vi "Telescope HK Data to Table.vi"(10 "Ch Info":T1[](array[typedef]), 11 "HK Data Cluster":T3) -> (3 "Table":string[][](array[string]))   [LabVIEW 2021, in "Telescope.lvclass"]
uses:
  Telescope.lvclass
  hk-channel-class/HK Item/HK Channel cluster Telemetry Data.ctl
  hk-channel-class/HK Item/HK Channel enum Data Type.ctl
  hk-channel-class/HK Item/HK Channel Units and Setup.ctl
  hk-channel-class/HK Item/HK Item.lvclass
panel:
  in  "Housekeeping Data":i32(listbox)
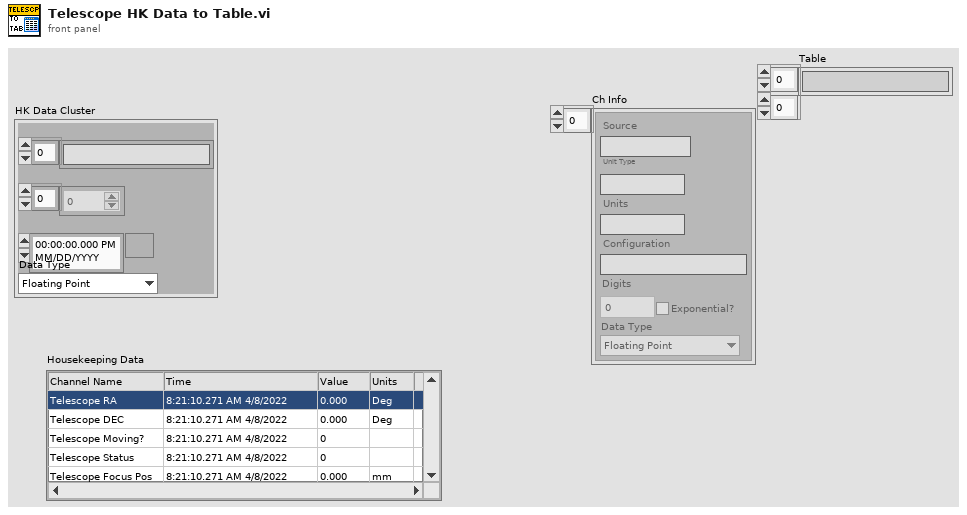
[diagram p1: front panel]
types:
  T1 = typedef "HK Item.lvclass/HK Channel Units and Setup.ctl" = cluster{"Unit Type":string, "Units":string, "Configuration":string, "Digits":i32, "Data Type":T2, "Exponential?":bool, "Source":string}
  T2 = typedef "HK Item.lvclass/HK Channel enum Data Type.ctl" = enum16{"Floating Point", "Integer", "Enum", "String", "Waveform", "File"}
  T3 = typedef "HK Item.lvclass/HK Channel cluster Telemetry Data.ctl" = cluster{"Ch Names":string[], "Ch Values":dbl[], "Timestamp":timestamp, "Data Type":T2}
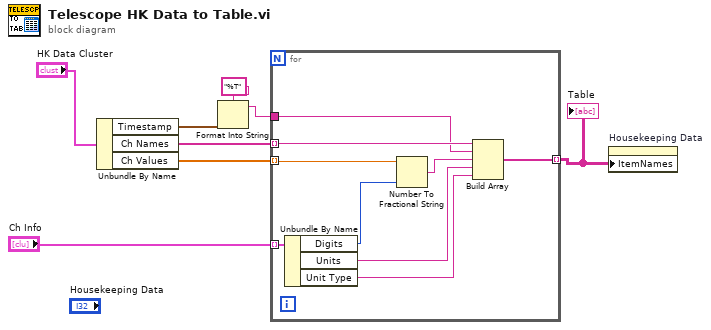
[diagram p0: block diagram]
diagram:
  n1 = Unbundle By Name("HK Data Cluster") -> ("Timestamp"=w3:timestamp, "Ch Names"=w7:string[], "Ch Values"=w6:dbl[])
  n2 = Format Into String(format string="%T", w3) -> (resulting string=w2:string)  [unwired: 2 in, 1 out]
  n3 = for {
    tunnel: w7 -> [w14] mode=indexing
    tunnel: w6 -> [w17] mode=indexing
    tunnel: "Ch Info" -> [w16] mode=indexing
    tunnel: w2 -> [w13]
    tunnel: [w10] -> w1 mode=indexing
    n4 = Unbundle By Name(w16) -> ("Digits"=w15:i32, "Units"=w11:string, "Unit Type"=w9:string)
    n5 = Number To Fractional String(number=w17, precision (6)=w15) -> (F-format string=w12:string)  [unwired: 2 in]
    n6 = Build Array(w14, w13, w12, w11, w9) -> (w10:string[])
  }
  "Table" <- w1
  n7 = property on="Housekeeping Data" class="MCListbox (strict)"("ItemNames"=w1) -> ()  [unwired: 2 in, 2 out]
